vi "Read DMM classes.vi"(11 "Measurements in":refnum<class "Measurement.lvclass">) -> (2 "DMM classes":refnum<class "Digital Multimeter.lvclass">[](array[class]), 3 "Measurements out":refnum<class "Measurement.lvclass">)   [LabVIEW 2020, in "Measurement.lvclass"]
uses:
  Measurement.lvclass
  Instruments/Digital Multimeter/Digital Multimeter.lvclass
  Measurement.lvclass/Measurement.ctl
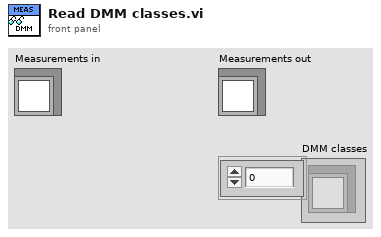
[diagram p1: front panel]
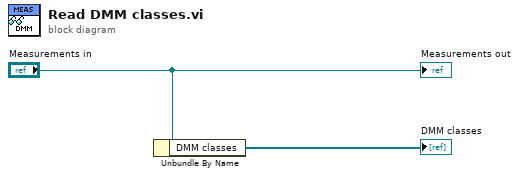
[diagram p0: block diagram]
diagram:
  n1 = Unbundle By Name("Measurements in") -> ("DMM classes"=→"DMM classes":refnum<class "Digital Multimeter.lvclass">[])
  "Measurements out" <- "Measurements in"
